vi "Receiver.vi"() -> ()   [LabVIEW 2014]
uses:
  CommState.ctl
panel:
  out "data out":dbl
  out "error out":errorcluster
  in  "stop":bool
  in  "IP Address":string="localhost"
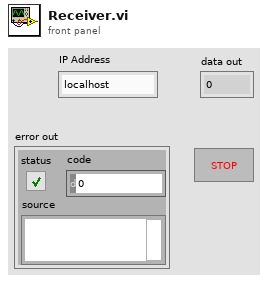
[diagram p1: front panel]
types:
  T1 = typedef "CommState.ctl" = enum16{"Disconnected", "Connected"}
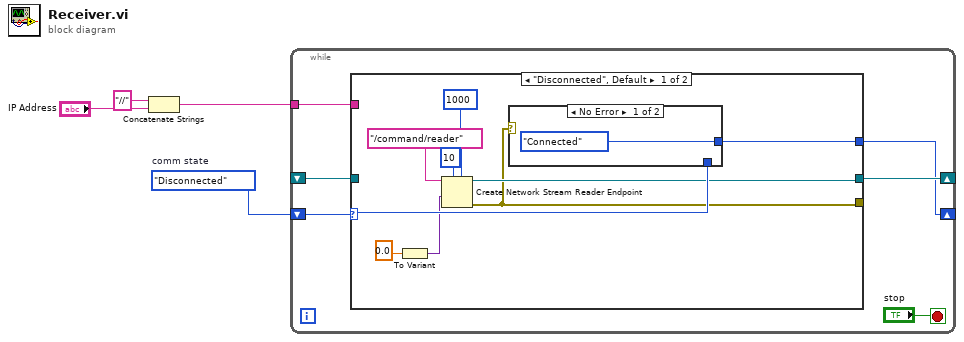
[diagram p0: block diagram]
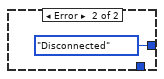
[diagram p2: hidden frame]
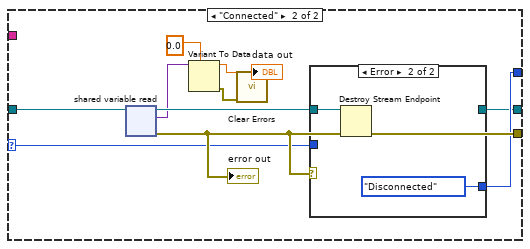
[diagram p3: hidden frame]
diagram:
  w4 = CommState."Disconnected"  # comm state
  n1 = Concatenate Strings("//" ("reader url"), "IP Address") -> (w1:string)
  n2 = while {
    tunnel: w1 -> [w9]
    shift-right: [w8] -> _
    shift-left: _ -> [w7]
    shift-right: [w5] -> _
    shift-left: w4 -> [w10]
    stop <- "stop" stop-if-true
    n3 = case shown="\"Disconnected\", Default" w10 {
      selector: w10 -> [w18 w29]
      tunnel: w9 -> [_ _]
      tunnel: [w15 w26] -> w8
      tunnel: w7 -> [_ w31]
      tunnel: [w14 w30] -> _
      tunnel: [w19 w28] -> w5
      frame "Disconnected", Default {
        n4 = To Variant(anything=0.0) -> (Variant=w12:variant)
        n5 = Create Network Stream Reader Endpoint(5:1000 ("timeout in ms (-1)"), 7:10 ("reader buffer size"), 9:w12, 11:"/command/reader" ("writer name")) -> (0:w14:errorcluster, 3:w15:refnum<k21>)  [unwired: 3 in]
        n6 = case shown="No Error" w14 {
          tunnel: [CommState."Connected" ("comm state") CommState."Disconnected" ("comm state")] -> w19
          tunnel: w18 -> [_ _]
          frame No Error {
          }
          frame Error {
          }
        }
      }
      frame "Connected" {
        n7 = shared-variable-read(w31) -> (w27:refnum<k21>, w30:errorcluster, w25:variant)  [unwired: 2 in, 1 out]
        "error out" <- w30
        n8 = Variant To Data(type=0.0, Variant=w25) -> (data=→"data out":dbl, error out=w22:errorcluster)  [unwired: 1 in]
        n9 = call <vilib>:"Clear Errors.vi"("error in (no error)"=w22) -> ()  [unwired: 5 in, 2 out]
        n10 = case shown="Error" w30 {
          tunnel: w29 -> [w33 _]
          tunnel: [w33 CommState."Disconnected" ("comm state")] -> w28
          tunnel: w27 -> [w32 w34]
          tunnel: [w32 _] -> w26
          frame No Error {
          }
          frame Error {
            n11 = Destroy Stream Endpoint(11:w34) -> ()  [unwired: 1 in, 1 out]
          }
        }
      }
    }
  }
